vi "svx_Polar_Set_Internal_States.vi"(9 "previous state":T2={"Property Name"=[], "Container bounds"={"Width"=550, "Height"=250}, "Scale range"={"Maximum"=1.0, "Increment"=1.0}, "PointIdx"=0, "Marker list"=[], "Color settings"={"Arrow color"=16860, "Magnitude major grid"=13816530, "Magnitude minor grid"=16777216, "Phase grid"=13816530, "Phase scale marker text"=0}, "Magnitude scale name"="Magnitude", "Magnitude scale format string"="%#.2e", "MagnitudeScale:Visible"=TRUE, "MagnitudeScaleLabel:Visible"=TRUE, "PhaseScale:Visible"=TRUE, "Marker:Visible"=TRUE, "Cursor:Visible"=FALSE, "CursorName:Visible"=TRUE, "Autoscale"=TRUE, "Marker color"=16860, "Line color"=16711680, "Cursor color"=16711680, "Magnitude scale marker color"=0, "Plot.Line Style"=0, "Plot.Line Width"=0, "Plot.Point Style"=0, "Cursor.Line Style"=0, "Cursor.Line Width"=0, "Cursor.Point Style"=0, "Cursor.Style"=4, "Marker.Point Style"=2, "Point/fill color"=16711680, "Background color"=16777225, "Cursor name"="", "Cursor Release"=refnum, "Scale Range Change"=refnum, "data size(s)"=[], "Selectors:Visible"=TRUE, "Selector:ring Strings"={"Selector:Custom Strings"=FALSE, "Selector:Row Strings []"=[], "Selector:Column Strings []"=[], "User:Row Strings []"=[], "User:Column Strings []"=[]}, "Lock Cursor Info Position"=FALSE, "CursLoc"={"magnitude"=0.0, "phase"=0.0, "time/rev/RPM"=0.0}, "Plot Area:Position"={"Left"=0, "Top"=0}, "Plot Area:Size"={"Width"=0, "Height"=0}, "Marker.Style"=0, "Indication Arcs"=[], "Arc.Selector"=0, "customized marker"=[], "tree Width"=0, " Parents Tags"=[], "Children Tags"=[], "open?"=[], "index"=[{"row index"=0, "column index"=0}], "Label"="", "custom strings changed"=FALSE, "Owning VI"=refnum, "Legend BG color"=16777225, "Legend font color"=0, "column Width"=203, "attribute"=variant} caption="State", 10 "current state":T2={"Property Name"=[], "Container bounds"={"Width"=550, "Height"=250}, "Scale range"={"Maximum"=1.0, "Increment"=1.0}, "PointIdx"=0, "Marker list"=[], "Color settings"={"Arrow color"=16860, "Magnitude major grid"=13816530, "Magnitude minor grid"=16777216, "Phase grid"=13816530, "Phase scale marker text"=0}, "Magnitude scale name"="Magnitude", "Magnitude scale format string"="%#.2e", "MagnitudeScale:Visible"=TRUE, "MagnitudeScaleLabel:Visible"=TRUE, "PhaseScale:Visible"=TRUE, "Marker:Visible"=TRUE, "Cursor:Visible"=FALSE, "CursorName:Visible"=TRUE, "Autoscale"=TRUE, "Marker color"=16860, "Line color"=16711680, "Cursor color"=16711680, "Magnitude scale marker color"=0, "Plot.Line Style"=0, "Plot.Line Width"=0, "Plot.Point Style"=0, "Cursor.Line Style"=0, "Cursor.Line Width"=0, "Cursor.Point Style"=0, "Cursor.Style"=4, "Marker.Point Style"=2, "Point/fill color"=16711680, "Background color"=16777225, "Cursor name"="", "Cursor Release"=refnum, "Scale Range Change"=refnum, "data size(s)"=[], "Selectors:Visible"=TRUE, "Selector:ring Strings"={"Selector:Custom Strings"=FALSE, "Selector:Row Strings []"=[], "Selector:Column Strings []"=[], "User:Row Strings []"=[], "User:Column Strings []"=[]}, "Lock Cursor Info Position"=FALSE, "CursLoc"={"magnitude"=0.0, "phase"=0.0, "time/rev/RPM"=0.0}, "Plot Area:Position"={"Left"=0, "Top"=0}, "Plot Area:Size"={"Width"=0, "Height"=0}, "Marker.Style"=0, "Indication Arcs"=[], "Arc.Selector"=0, "customized marker"=[], "tree Width"=0, " Parents Tags"=[], "Children Tags"=[], "open?"=[], "index"=[{"row index"=0, "column index"=0}], "Label"="", "custom strings changed"=FALSE, "Owning VI"=refnum, "Legend BG color"=16777225, "Legend font color"=0, "column Width"=203, "attribute"=variant} caption="State", 11 "state":T1) -> (3 "state out":T1)   [LabVIEW 2017, in "SVX Polar Plot.xctl"]
uses:
  <vilib>/addons/_XControls/Polar Plot/SVX Polar Plot.xctl
  <vilib>/addons/_XControls/Polar Plot/subVIs/svx_Polar_Plot_State.ctl
  <vilib>/addons/_XControls/Polar Plot/subVIs/svx_Polar_Plot_Internal_State.ctl
  <vilib>/addons/_XControls/Polar Plot/subVIs/svx_Polar_Indication_Arcs.ctl
  <vilib>/addons/_XControls/Polar Plot/subVIs/svx_Polar_Customized_Markers.ctl
panel:
  out "timed out?":bool
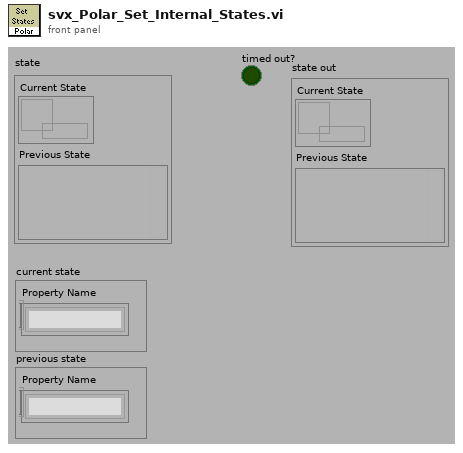
[diagram p1: front panel]
types:
  T1 = typedef "SVX Polar Plot.xctl/svx_Polar_Plot_State.ctl" = cluster{"Current State":refnum<queue>, "Previous State":variant}
  T2 = typedef "SVX Polar Plot.xctl/svx_Polar_Plot_Internal_State.ctl" = cluster{"Property Name":string[], "Container bounds":cluster{"Width":u32, "Height":u32}, "Scale range":cluster{"Maximum":dbl, "Increment":dbl}, "PointIdx":i32, "Marker list":cluster{"Name":string, "Color":u32, "Style":u8, "Point Style":u8, "Name Visible":bool, "Allow Drag":bool, "Annotation Mode":u32, "Plot":i32, "Index":i32, "Position":cluster{"X":dbl, "Y":dbl}, "X Scale":u32, "Y Scale":u32, "Show Arrow":bool, "Lock Name":bool, "Plot Area":i32, "Label Offset":cluster{"X":dbl, "Y":dbl}}[], "Color settings":cluster{"Arrow color":u32, "Magnitude major grid":u32, "Magnitude minor grid":u32, "Phase grid":u32, "Phase scale marker text":u32}, "Magnitude scale name":string, "Magnitude scale format string":string, "MagnitudeScale:Visible":bool, "MagnitudeScaleLabel:Visible":bool, "PhaseScale:Visible":bool, "Marker:Visible":bool, "Cursor:Visible":bool, "CursorName:Visible":bool, "Autoscale":bool, "Marker color":u32, "Line color":u32, "Cursor color":u32, "Magnitude scale marker color":u32, "Plot.Line Style":i32, "Plot.Line Width":i32, "Plot.Point Style":i32, "Cursor.Line Style":i32, "Cursor.Line Width":i32, "Cursor.Point Style":i32, "Cursor.Style":i32, "Marker.Point Style":i32, "Point/fill color":u32, "Background color":u32, "Cursor name":string, "Cursor Release":refnum<user-event>, "Scale Range Change":refnum<user-event>, "data size(s)":i32[], "Selectors:Visible":bool, "Selector:ring Strings":cluster{"Selector:Custom Strings":bool, "Selector:Row Strings []":string[], "Selector:Column Strings []":string[], "User:Row Strings []":string[], "User:Column Strings []":string[]}, "Lock Cursor Info Position":bool, "CursLoc":cluster{"magnitude":dbl, "phase":dbl, "time/rev/RPM":dbl}, "Plot Area:Position":cluster{"Left":i32, "Top":i32}, "Plot Area:Size":cluster{"Width":u32, "Height":u32}, "Marker.Style":i32, "Indication Arcs":T3, "Arc.Selector":u16, "customized marker":T4, "tree Width":u32, " Parents Tags":string[], "Children Tags":string[], "open?":bool[], "index":cluster{"row index":i32, "column index":i32}[], "Label":string, "custom strings changed":bool, "Owning VI":refnum<vi>, "Legend BG color":u32, "Legend font color":u32, "column Width":u32, "attribute":variant}
  T3 = typedef "SVX Polar Plot.xctl/svx_Polar_Indication_Arcs.ctl" = cluster{"Name":string, "Start radius":dbl, "End radius":dbl, "Line Style":i32, "Line Width":i32, "Border color":u32, "Fill color":u32, "Start angle":i16, "End angle":i16, "Visible":bool}[]
  T4 = typedef "SVX Polar Plot.xctl/svx_Polar_Customized_Markers.ctl" = cluster{"Name":string, "Color":u32, "Style":u8, "Point Style":u8, "Name Visible":bool, "Allow Drag":bool, "Annotation Mode":u32, "Plot":i32, "Index":i32, "Position":cluster{"Magnitude":dbl, "Phase":dbl}, "X Scale":u32, "Y Scale":u32, "Show Arrow":bool, "Lock Name":bool, "Plot Area":i32, "Label Offset":cluster{"Magnitude":dbl, "Phase":dbl}}[]
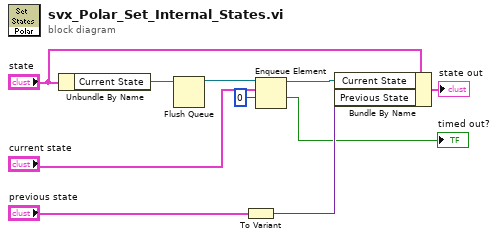
[diagram p0: block diagram]
diagram:
  n1 = Unbundle By Name("state") -> ("Current State"=w2:refnum<queue>)
  n2 = Flush Queue(queue=w2) -> (queue out=w1:refnum<queue>)  [unwired: 1 in, 2 out]
  n3 = To Variant(anything="previous state") -> (Variant=w6:variant)
  n4 = Enqueue Element(queue=w1, element="current state", timeout in ms (-1)=0) -> (queue out=w8:refnum<queue>, timed out?=→"timed out?":bool)  [unwired: 1 in, 1 out]
  n5 = Bundle By Name(cluster="state", "Current State"=w8, "Previous State"=w6) -> (→"state out":T1)
